vi "CaptureImage2.vi"(10 "FileName":string="andre", 11 "VISA resource name":refnum<visa-resource-name>="COM5") -> (0 "error out":errorcluster, 2 "success?":bool=TRUE, 3 "ImageFilepath":path)   [LabVIEW 2014]
panel:
  out "Receive Buffer_MP":u8[](array[numeric])
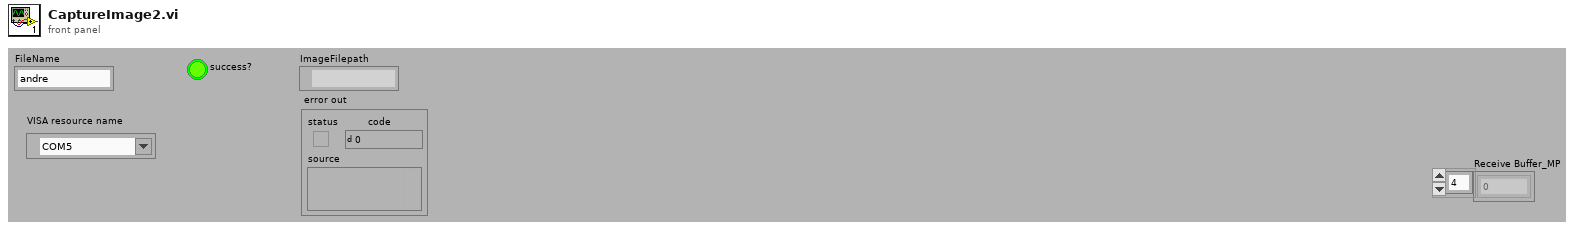
[diagram p1: front panel]
types:
  T1 = enum16{"Enter FAT", "Beeper Control", "LED Off", "LED On", "Image Mode", "Start Session", "Stop Session", "Change Buadrate", "Auto Exposure", "Set Manual Exposure", "Read BT Address", "Store BT Address", "Pairing Command", "Query Paired Address", "Pairing Status", "Un-Pairing", "Set Illumination", "Trigger", "Set Defaults", "Imager Time To Decode Test", "Battery Off", "Battery Charge Control", "Read Battery Voltage", "Read Battery Temperature", "Software Version", "StoreFeatureSet", "ReadFeatureSet", "Store Model Number", "Read Model Number", "Store Manufacturing Date", "Read Manufacturing Date", "Store Service Date", "Read Service Date", "Store Serial Number", "Read Serial Number", "Exit FAT", "Read GUID", "Cable Auto ID", "Store RSM 627", "Read RSM 627", "Hall Effect switch", "Store GUID "}
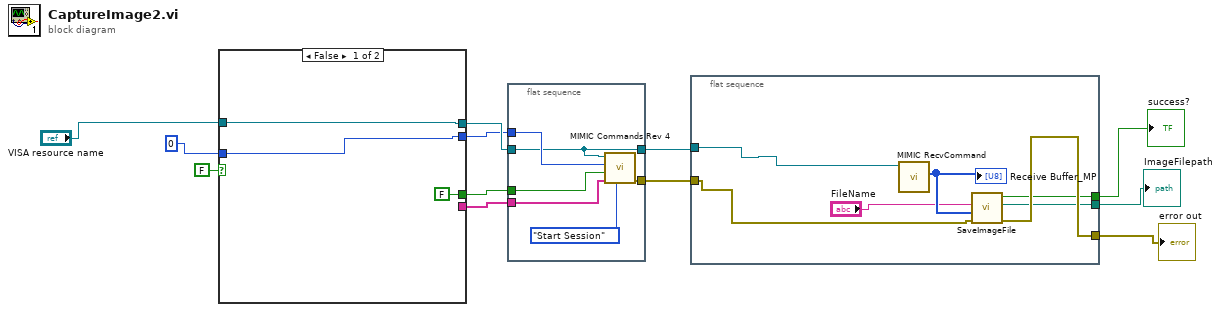
[diagram p0: block diagram]
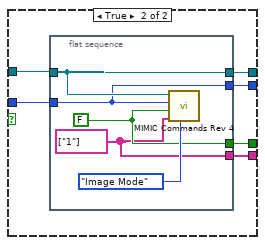
[diagram p2: hidden frame]
diagram:
  n1 = case shown="False" FALSE {
    tunnel: [w15 w21] -> w11
    tunnel: u32 0 ("wait (ms)") -> [w14 w20]
    tunnel: [w14 w19] -> w9
    tunnel: [FALSE ("HWHSflag") w18] -> w8
    tunnel: [_ w17] -> w7
    tunnel: "VISA resource name" -> [w15 w16]
    frame False {
    }
    frame True {
      n2 = flat-sequence {
        tunnel: w16 -> [w25]
        tunnel: [w25] -> w21
        tunnel: w20 -> [w24]
        tunnel: [w24] -> w19
        tunnel: [w23] -> w18
        tunnel: [w22] -> w17
        frame #0 {
          w22 = string[] ["1"] ("Input String Data Array")
          w23 = FALSE ("HWHSflag")
          n3 = call "MIMIC Commands Rev 4.vi"("MIMIC HOST COMMAND"=T1."Image Mode", "Input String Data Array"=w22, "HWHSflag"=w23, "wait (ms)"=w24, "VISA resource name"=w25) -> ()  [unwired: 4 in, 3 out]
        }
      }
    }
  }
  n4 = flat-sequence {
    tunnel: w7 -> [w31]
    tunnel: w8 -> [w30]
    tunnel: w9 -> [w29]
    tunnel: w11 -> [w28]
    tunnel: [w28] -> w12
    tunnel: [w27] -> w2
    frame #0 {
      n5 = call "MIMIC Commands Rev 4.vi"("MIMIC HOST COMMAND"=T1."Start Session", "Input String Data Array"=w31, "HWHSflag"=w30, "wait (ms)"=w29, "VISA resource name"=w28) -> ("error out"=w27:errorcluster)  [unwired: 4 in, 2 out]
    }
  }
  n6 = flat-sequence {
    tunnel: w12 -> [w38]
    tunnel: [w36] -> w4
    tunnel: [w35] -> w3
    tunnel: w2 -> [w34]
    tunnel: [w33] -> w1
    frame #0 {
      n7 = call "MIMIC RecvCommand.vi"("VISA resource name"=w38) -> ("Receive Buffer_MP"=w39:u8[])  [unwired: 3 in, 3 out]
      "Receive Buffer_MP" <- w39
      n8 = call "SaveImageFile.vi"("error in"=w34, "ImagData"=w39, "FileName"="FileName") -> ("error out"=w36:errorcluster, "appended path"=w35:path, "success?"=w33:bool)  [unwired: 6 in]
    }
  }
  "error out" <- w4
  "ImageFilepath" <- w3
  "success?" <- w1
